vi "Multi Dut Cmd VPI Setting.vi"(8 "error in (no error)":errorcluster, 10 "Cmin/Act":bool=TRUE, 11 "WS1050/51":bool=TRUE) -> (0 "error out":errorcluster, 1 "Cmd VPI C3":string[](array[string]), 2 "VPI_C3":string[](array[string]), 3 "Name Header VPI":string[](array[string]), 4 "Cmd VPI C2":string[](array[string]), 5 "VPI_C2":string[](array[string]), 6 "Cmd VPI C1":string[](array[string]), 7 "VPI_C1":string[](array[string]))   [LabVIEW 2012]
panel:
  in  "VPI_Cmd 51 Cmin":string[](array[string])=["00", "00", "00"]
  in  "VPI_Cmd 50 Cmin":string[](array[string])=["00", "00", "00"]
  in  "VPI_Cmd 51":string[](array[string])=["00", "2F", "00"]
  in  "VPI Name 51":string[](array[string])=["All_Drivers OFF", "All Drivers ON", "All Drivers OFF2"]
  in  "VPI_Cmd 50":string[](array[string])=["00", "3B", "00"]
  in  "VPI Name 50":string[](array[string])=["All_Drivers OFF", "All Drivers ON", "All Drivers OFF2"]
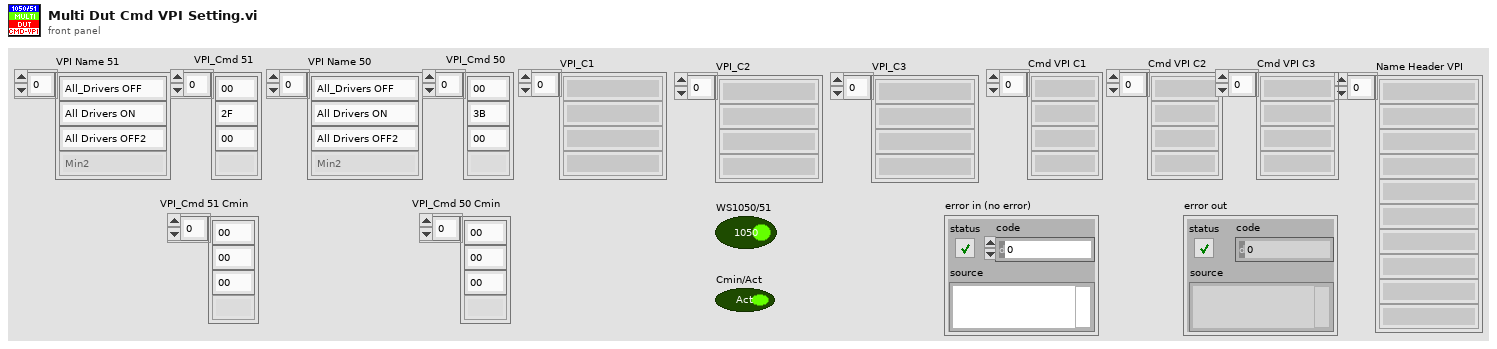
[diagram p1: front panel]
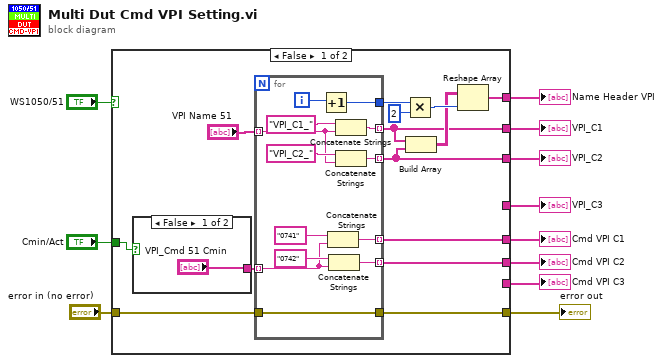
[diagram p0: block diagram]
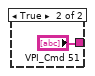
[diagram p2: hidden frame]
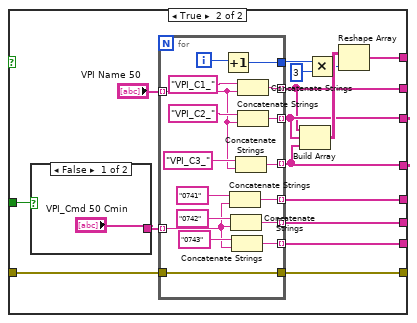
[diagram p3: hidden frame]
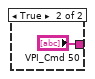
[diagram p4: hidden frame]
diagram:
  n1 = case shown="False" "WS1050/51" {
    tunnel: "error in (no error)" -> [w17 w50]
    tunnel: [w18 w49] -> w9
    tunnel: [w19 w48] -> w8
    tunnel: [w15 w47] -> w7
    tunnel: [w16 w46] -> w6
    tunnel: [_ w45] -> w5
    tunnel: [w14 w44] -> w4
    tunnel: [w13 w43] -> w3
    tunnel: [_ w42] -> w2
    tunnel: "Cmin/Act" -> [w12 w41]
    frame False {
      n2 = case shown="False" w12 {
        tunnel: ["VPI_Cmd 51 Cmin" "VPI_Cmd 51"] -> w21
        frame False {
        }
        frame True {
        }
      }
      n3 = for {
        tunnel: "VPI Name 51" -> [w29] mode=indexing
        tunnel: w21 -> [w34] mode=indexing
        tunnel: [w38] -> w16 mode=indexing
        tunnel: [w37] -> w15 mode=indexing
        tunnel: [w33] -> w14 mode=indexing
        tunnel: [w32] -> w13 mode=indexing
        tunnel: [w30] -> w23
        tunnel: w17 -> [w28]
        tunnel: [w28] -> w18
        i -> [w31]
        n4 = Increment(x=w31) -> (x+1=w30:i32)
        n5 = Concatenate Strings("0741" ("string"), w34) -> (w33:string)
        n6 = Concatenate Strings("0742" ("string"), w34) -> (w32:string)
        n7 = Concatenate Strings("VPI_C1_" ("string"), w29) -> (w38:string)
        n8 = Concatenate Strings("VPI_C2_" ("string"), w29) -> (w37:string)
      }
      n9 = Multiply(x=w23, y=2) -> (x*y=w24:i32)
      n10 = Build Array(w16, w15) -> (w22:string[][])
      n11 = Reshape Array(w22, w24) -> (w19:string[])
    }
    frame True {
      n12 = case shown="False" w41 {
        tunnel: ["VPI_Cmd 50 Cmin" "VPI_Cmd 50"] -> w55
        frame False {
        }
        frame True {
        }
      }
      n13 = for {
        tunnel: "VPI Name 50" -> [w60] mode=indexing
        tunnel: w55 -> [w66] mode=indexing
        tunnel: [w72] -> w46 mode=indexing
        tunnel: [w71] -> w47 mode=indexing
        tunnel: [w70] -> w45 mode=indexing
        tunnel: [w65] -> w44 mode=indexing
        tunnel: [w64] -> w43 mode=indexing
        tunnel: [w63] -> w42 mode=indexing
        tunnel: [w61] -> w53
        tunnel: w50 -> [w59]
        tunnel: [w59] -> w49
        i -> [w62]
        n14 = Increment(x=w62) -> (x+1=w61:i32)
        n15 = Concatenate Strings("0741" ("string"), w66) -> (w65:string)
        n16 = Concatenate Strings("0742" ("string"), w66) -> (w64:string)
        n17 = Concatenate Strings("0743" ("string"), w66) -> (w63:string)
        n18 = Concatenate Strings("VPI_C3_" ("string"), w60) -> (w70:string)
        n19 = Concatenate Strings("VPI_C1_" ("string"), w60) -> (w72:string)
        n20 = Concatenate Strings("VPI_C2_" ("string"), w60) -> (w71:string)
      }
      n21 = Build Array(w46, w47, w45) -> (w54:string[][])
      n22 = Multiply(x=w53, y=3) -> (x*y=w52:i32)
      n23 = Reshape Array(w54, w52) -> (w48:string[])
    }
  }
  "error out" <- w9
  "Name Header VPI" <- w8
  "VPI_C2" <- w7
  "VPI_C1" <- w6
  "VPI_C3" <- w5
  "Cmd VPI C1" <- w4
  "Cmd VPI C2" <- w3
  "Cmd VPI C3" <- w2
